vi "Power Line Frequency Conversion.vi"(0 "Power line frequency":T1 items=["50 Hz", "60 Hz"]) -> (4 "Power Line Freq":dbl)   [LabVIEW 2024, in "devicePowerSequencerCoreLogic.lvlib"]
uses:
  devicePowerSequencerCoreLogic.lvlib
  controls/Power line frequency.ctl
  Device Power Sequencer.lvlib
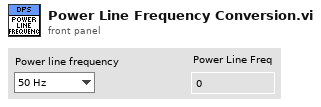
[diagram p1: front panel]
types:
  T1 = typedef "Device Power Sequencer.lvlib/Power line frequency.ctl" = u32
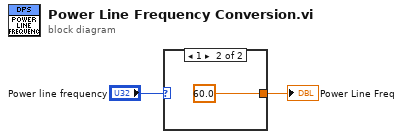
[diagram p0: block diagram]
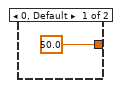
[diagram p2: hidden frame]
diagram:
  n1 = case shown="1" "Power line frequency" {
    tunnel: [50.0 ("Power Line Freq") 60.0 ("Power Line Freq")] -> w1
    frame 0, Default {
    }
    frame 1 {
    }
  }
  "Power Line Freq" <- w1
